vi "IFNoise-Create Stimulus.vi"(0 "Path":path, 7 "InvFilt Params":T2={"Min Frequency (Hz)"=0.0, "Max Frequency (Hz)"=0.0, "Length (points)"=301, "Sampling rate (Hz)"=0.0, "Delay (ms)"=301.0, "Linear phase"=FALSE}, 11 "error in (no error)":errorcluster, 12 "Inverse Filter":bool) -> (3 "Mag Spec":T1, 4 "Noise":dbl[](array[numeric]), 14 "Max SPL":dbl, 15 "error out":errorcluster)   [LabVIEW 2015]
uses:
  Inverse Filter VIs/InvFilt-Params.ctl
  <vilib>/Analysis/5stat.llb/RMS (DBL).vi
  PXI DAQ VIs/DAQ Engine VIs/PXI Globals.vi
  Utility VIs/Math VIs/Linear to dB (scalar).vi
  <vilib>/Analysis/NI_AALBase.lvlib
  <vilib>/Analysis/NI_AALPro.lvlib
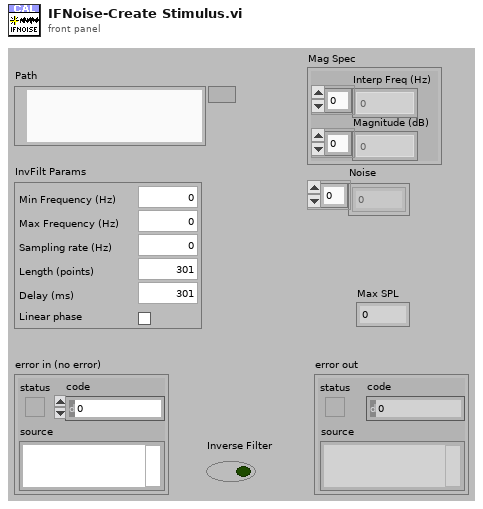
[diagram p1: front panel]
types:
  T1 = cluster{"Interp Freq (Hz)":dbl[], "Magnitude (dB)":dbl[]}
  T2 = typedef "InvFilt-Params.ctl" = cluster{"Min Frequency (Hz)":dbl, "Max Frequency (Hz)":dbl, "Length (points)":i32, "Sampling rate (Hz)":dbl, "Delay (ms)":dbl, "Linear phase":bool}
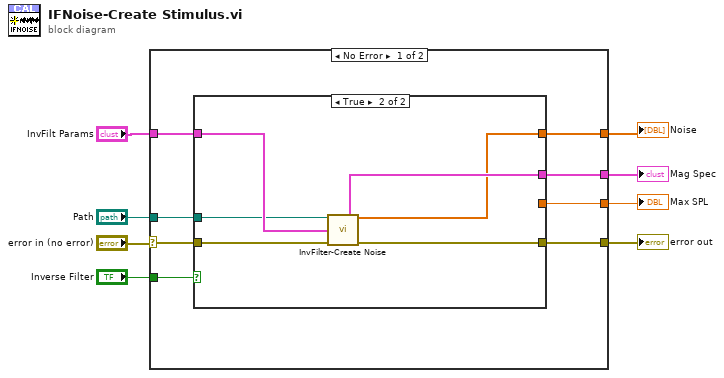
[diagram p0: block diagram]
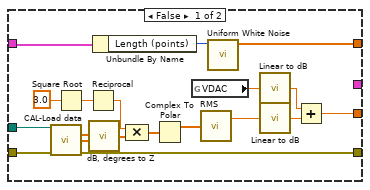
[diagram p2: hidden frame]
diagram:
  n1 = case shown="No Error" "error in (no error)" {
    selector: "error in (no error)" -> [w15 w42]
    tunnel: [w10 w42] -> w7
    tunnel: "Inverse Filter" -> [w16 _]
    tunnel: "InvFilt Params" -> [w14 _]
    tunnel: "Path" -> [w13 _]
    tunnel: [w12 _] -> w3
    tunnel: [w11 _] -> w2
    tunnel: [w9 _] -> w1
    frame No Error {
      n2 = case shown="True" w16 {
        tunnel: w15 -> [w22 w41]
        tunnel: w14 -> [w35 w40]
        tunnel: w13 -> [w23 w39]
        tunnel: [_ w38] -> w12
        tunnel: [w33 w37] -> w11
        tunnel: [w21 w36] -> w10
        tunnel: [w17 _] -> w9
        frame False {
          n3 = call "CAL-Load data.vi"("user path"=w23, "error in (no error)"=w22) -> ("Mag"=w30:dbl[], "Phase"=w29:dbl[], "error out"=w21:errorcluster)  [unwired: 6 in, 5 out]
          n4 = Square Root(x=3.0 ("Noise Vrms")) -> (sqrt(x)=w19:dbl)
          n5 = Reciprocal(x=w19) -> (1/x=w18:dbl)
          n6 = call "dB, degrees to Z.vi"("Magnitude (dB)"=w30, "Phase (degrees)"=w29) -> ("Z"=w26:cdb[])  [unwired: 5 in]
          n7 = Unbundle By Name(w35) -> ("Length (points)"=w34:i32)
          n8 = Compound Arithmetic op=MULTIPLY(w18, w26) -> (w27:cdb[])
          n9 = Complex To Polar(r * e^(i*theta)=w27) -> (r=w25:dbl[])  [unwired: 1 out]
          n10 = global read "PXI Globals.vi" "VDAC"() -> (w32:dbl)
          n11 = call-poly <vilib>:"RMS.vi"("X"=w25) -> ("rms value"=w28:dbl)  [unwired: 1 out]
          n12 = call <vilib>:"Uniform White Noise.vi"("samples"=w34) -> ("uniform white noise"=w33:dbl[])  [unwired: 9 in, 1 out]
          n13 = call-poly "Linear to dB.vi"("Linear"=w32) -> ("dB"=w31:dbl)
          n14 = call-poly "Linear to dB.vi"("Linear"=w28) -> ("dB"=w24:dbl)
          n15 = Add(x=w31, y=w24) -> (x+y=w17:dbl)
        }
        frame True {
          n16 = call "InvFilter-Create Noise.vi"("Calibration File"=w39, "InvFilt Params"=w40, "error in (no error)"=w41) -> ("Mag Spec"=w38:T1, "InvFilter Noise"=w37:dbl[], "error out"=w36:errorcluster)  [unwired: 9 in, 1 out]
        }
      }
    }
    frame Error {
    }
  }
  "error out" <- w7
  "Mag Spec" <- w3
  "Noise" <- w2
  "Max SPL" <- w1
